vi "Data Queue PtByPt.vi"(6 "initial queue element":dbl, 7 "initialize":bool, 10 "sample length":i32=100, 11 "input data point":dbl format="%0.2f") -> (0 "error":i32, 1 "Previous Queue":dbl[](array[numeric]), 2 "Current Queue":dbl[](array[numeric]), 3 "eliminated element":dbl format="%0.2f", 4 "current length":i32)   [LabVIEW 2017, in "NI_PtbyPt.lvlib"]
doc: "Creates a data queue of real numbers."
uses:
  <vilib>/ptbypt/NI_PtbyPt.lvlib
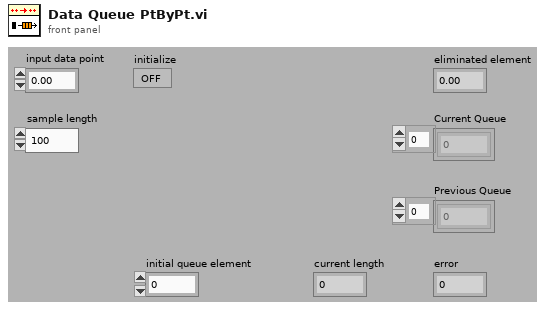
[diagram p1: front panel]
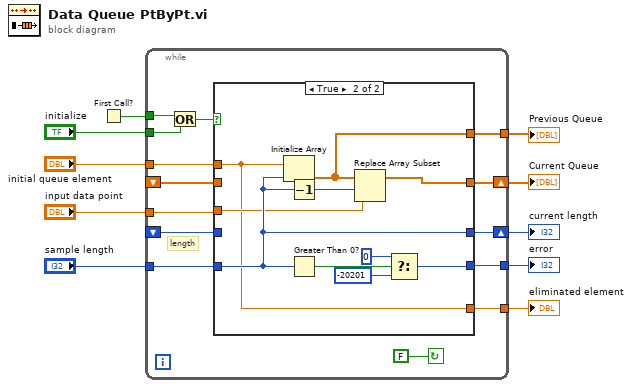
[diagram p0: block diagram]
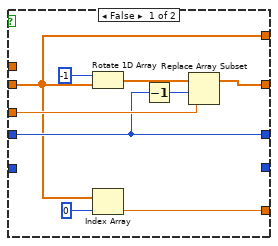
[diagram p2: hidden frame]
diagram:
  n1 = First Call?() -> (First Call?: T/F=w8:bool)
  n2 = while {
    tunnel: [w17] -> w7
    tunnel: w8 -> [w19]
    shift-left: _ -> [w22]
    shift-right: [w23] -> w9
    shift-left: _ -> [w21]
    shift-right: [w24] -> w10
    tunnel: "initialize" -> [w16]
    tunnel: "input data point" -> [w15]
    tunnel: "initial queue element" -> [w14]
    tunnel: "sample length" -> [w13]
    tunnel: [w12] -> w2
    tunnel: [w11] -> w1
    stop <- FALSE continue-if-true
    # "length"
    n3 = Or(x=w19, y=w16) -> (x .or. y?=w18:bool)
    n4 = case shown="True" w18 {
      tunnel: [w30 w36] -> w24
      tunnel: [w31 w39] -> w23
      tunnel: w22 -> [w31 _]
      tunnel: w21 -> [w27 _]
      tunnel: w15 -> [w32 w37]
      tunnel: [w27 w38] -> w17
      tunnel: w14 -> [_ w34]
      tunnel: w13 -> [_ w39]
      tunnel: [w25 w34] -> w12
      tunnel: [_ w35] -> w11
      frame False {
        n5 = Rotate 1D Array(1:w27, 2:i16 -1 ("n")) -> (0:w28:dbl[])
        n6 = Index Array(array=w27, index=0 ("Index")) -> (element=w25:dbl)
        n7 = Decrement(x=w31) -> (x-1=w29:i32)
        n8 = Replace Array Subset(array=w28, new element=w32, index=w29) -> (w30:dbl[])
      }
      frame True {
        n9 = Initialize Array(w34, w39) -> (w38:dbl[])
        n10 = Decrement(x=w39) -> (x-1=w43:i32)
        n11 = Greater Than 0?(x=w39) -> (x > 0?=w42:bool)
        n12 = Replace Array Subset(array=w38, new element=w37, index=w43) -> (w36:dbl[])
        n13 = Select(t=0, s=w42, f=-20201) -> (s? t:f=w35:i32)
      }
    }
  }
  "Current Queue" <- w10
  "current length" <- w9
  "Previous Queue" <- w7
  "eliminated element" <- w2
  "error" <- w1
